vi "load e-series.vi"(8 "error in (no error)":errorcluster, 11 "INI File":string) -> (0 "error out":errorcluster, 3 "E-Series Data":T1)   [LabVIEW 2018, in "E-Series Reader.lvlib"]
uses:
  E-Series Reader.lvlib
  series data--cluster.ctl
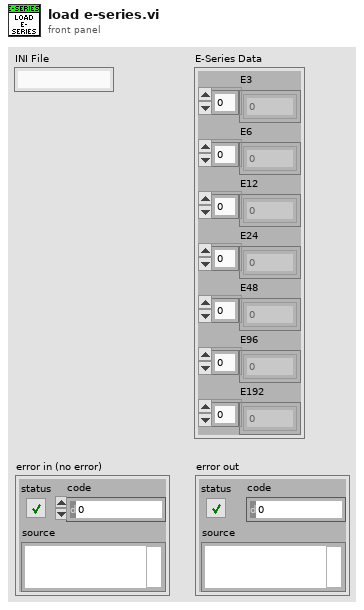
[diagram p1: front panel]
types:
  T1 = typedef "E-Series Reader.lvlib/series data--cluster.ctl" = cluster{"E3":u16[], "E6":u16[], "E12":u16[], "E24":u16[], "E48":u16[], "E96":u16[], "E192":u16[]}
  T2 = typedef "E-Series Reader.lvlib/e-series file names--array.ctl" = string[]
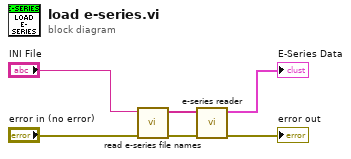
[diagram p0: block diagram]
diagram:
  n1 = call "read e-series file names.vi"("error in (no error)"="error in (no error)", "INI File"="INI File") -> ("error out"=w4:errorcluster, "E-Series File Names"=w3:T2)  [unwired: 8 in]
  n2 = call "e-series reader.vi"("error in"=w4, "E-Series File Names"=w3) -> ("error out"=→"error out":errorcluster, "E-Series Data"=→"E-Series Data":T1)  [unwired: 8 in]
